vi "convert abs chan num.vi"(0 "Abs Channel":i32, 5 "error in":errorcluster) -> (12 "num channels":i32, 13 "num pages":i32, 14 "Card type":string, 15 "Slot num":i32, 16 "set page":i32, 17 "Channel number in card":i32, 18 "Crate Num":i32, 19 "error out":errorcluster)   [LabVIEW 2018]
uses:
  CAEN globals.vi
panel:
  out "Card num of type":i32
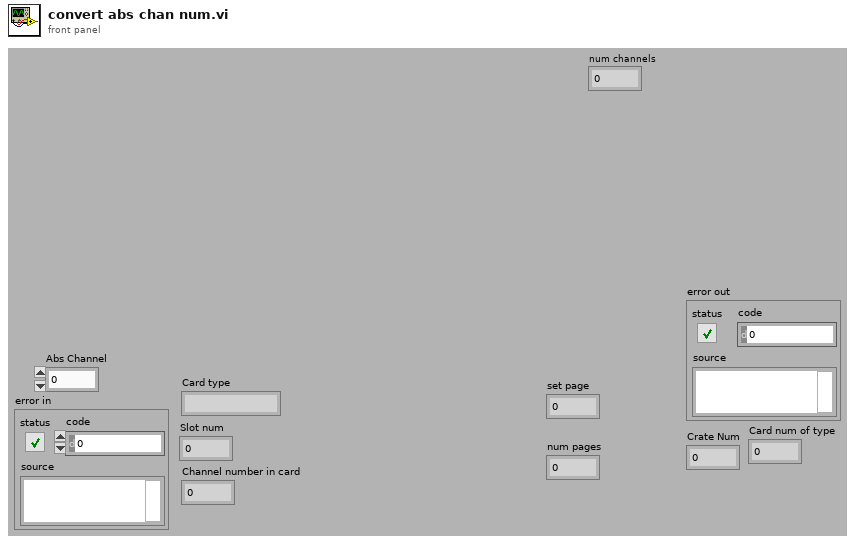
[diagram p1: front panel]
types:
  T1 = typedef "crate.ctl" = cluster{"CAENet Address":i32, "Crate Model":string, "Firmware Version":string, "Crate Map":T2[], "Total Channels":i32}
  T2 = typedef "card.ctl" = cluster{"Slot Number":i32, "Card Model":string, "Num Channels":i32, "Polarity":string, "Vmax":dbl, "Imax":dbl, "Revision":string}
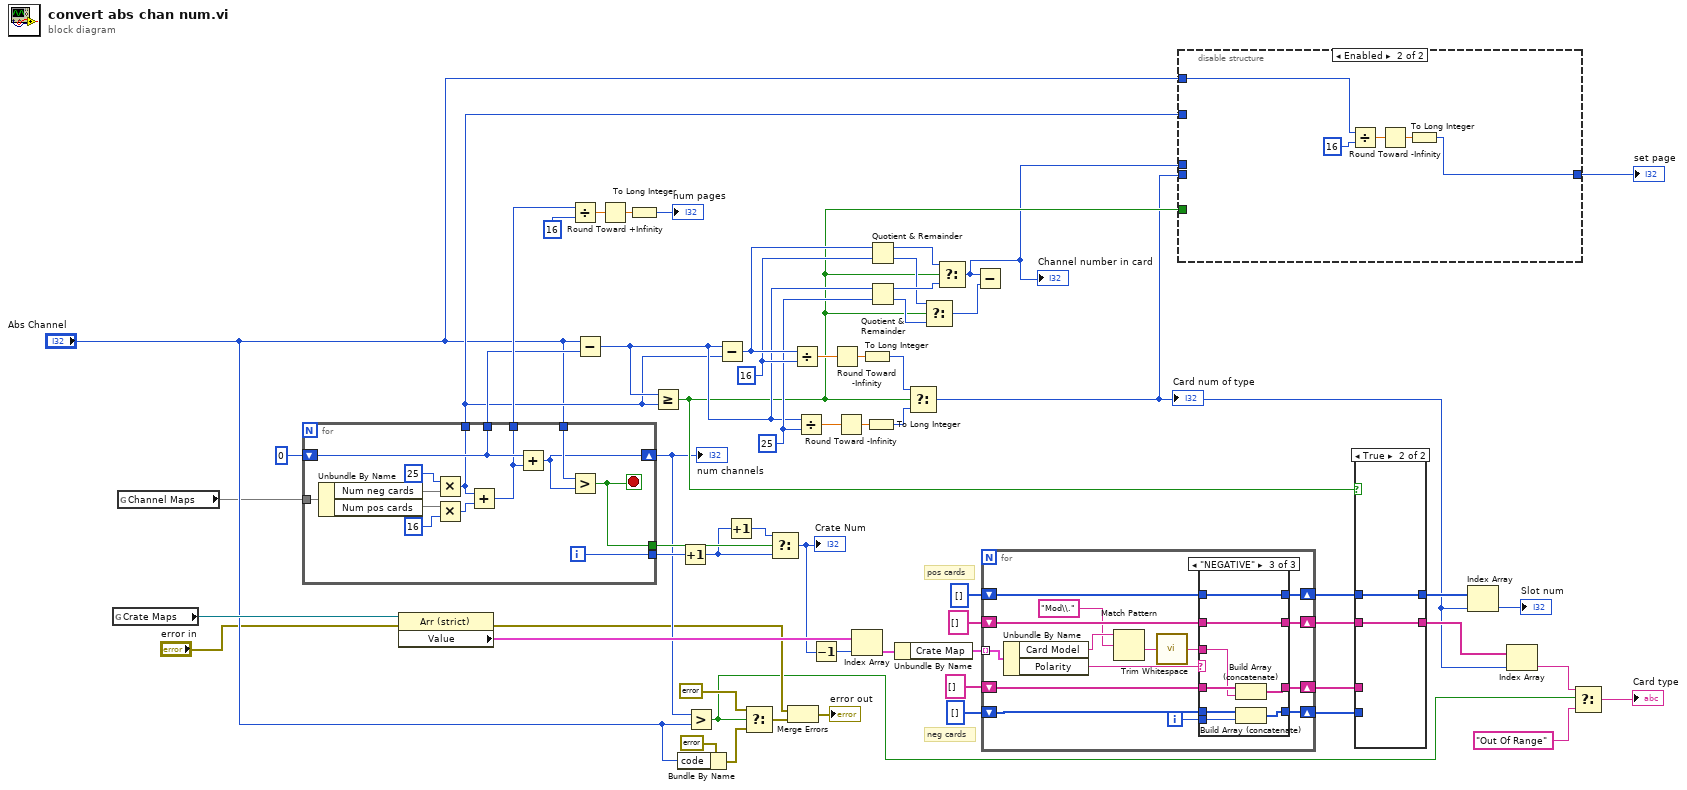
[diagram p0: block diagram]
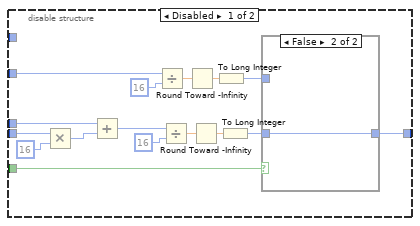
[diagram p2: hidden frame]
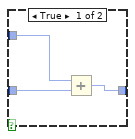
[diagram p3: hidden frame]
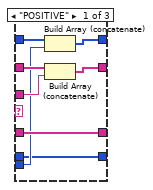
[diagram p5: hidden frame]
diagram:
  w54 = 25 ("y")
  w55 = 16 ("y")
  # "neg cards"
  # "pos cards"
  n1 = global read "CAEN globals.vi" "Crate Maps"() -> (w45:refnum<vi>)
  n2 = global read "CAEN globals.vi" "Channel Maps"() -> (w2)
  n3 = for {
    tunnel: w2 -> [w73]
    shift-right: [w68] -> w11
    shift-left: 0 -> [w67]
    tunnel: "Abs Channel" -> [w69]
    tunnel: [w65] -> w47
    tunnel: [w67] -> w20
    tunnel: [w66] -> w19
    tunnel: [w64] -> w49
    tunnel: [w63] -> w27
    i -> [w65]
    stop <- w64 stop-if-true
    n4 = Unbundle By Name(w73) -> ("Num neg cards"=w75, "Num pos cards"=w71)
    n5 = Multiply(x=25 ("y"), y=w75) -> (x*y=w66:i32)
    n6 = Multiply(x=w71, y=16) -> (x*y=w70:i32)
    n7 = Add(x=w66, y=w70) -> (x+y=w63:i32)
    n8 = Add(x=w67, y=w63) -> (x+y=w68:i32)
    n9 = Greater?(x=w69, y=w68) -> (0:w64:bool)
  }
  "num channels" <- w11
  n10 = property class="Arr (strict)"(reference=w45, error in="error in") -> (error out=w9:errorcluster, "Value"=w44:T1[])  [unwired: 1 out]
  n11 = Divide(x=w27, y=16) -> (x/y=w29:dbl)
  n12 = Subtract(x="Abs Channel", y=w20) -> (x-y=w51:i32)
  n13 = Round Toward +Infinity(x=w29) -> (ceil(x): smallest int >= x=w30:dbl)
  n14 = To Long Integer(number=w30) -> (32bit integer=→"num pages":i32)
  n15 = Greater Or Equal?(x=w51, y=w19) -> (x >= y?=w23:bool)
  n16 = Bundle By Name(cluster=errorcluster {"status"=TRUE, "code"=0, "source"="Channel out of range"} ("error out"), "code"="Abs Channel") -> (w15:errorcluster)
  n17 = Increment(x=w47) -> (x+1=w46:i32)
  n18 = Greater?(x=w11, y="Abs Channel") -> (0:w3:bool)
  n19 = Subtract(x=w51, y=w19) -> (x-y=w56:i32)
  n20 = Increment(x=w46) -> (x+1=w48:i32)
  n21 = Select(t=errorcluster {"status"=FALSE, "code"=0, "source"=""}, s=w3, f=w15) -> (s? t:f=w13:errorcluster)
  n22 = Select(t=w48, s=w49, f=w46) -> (s? t:f=w43:i32)
  "Crate Num" <- w43
  n23 = Merge Errors(w9, w13) -> (→"error out":errorcluster)
  n24 = Divide(x=w56, y=w55) -> (x/y=w57:dbl)
  n25 = Divide(x=w51, y=w54) -> (x/y=w61:dbl)
  n26 = Decrement(x=w43) -> (x-1=w42:i32)
  n27 = Round Toward -Infinity(1:w57) -> (0:w58:dbl)
  n28 = Round Toward -Infinity(1:w61) -> (0:w60:dbl)
  n29 = Index Array(array=w44, index=w42) -> (element=w41:T1)
  n30 = To Long Integer(number=w58) -> (32bit integer=w59:i32)
  n31 = To Long Integer(number=w60) -> (32bit integer=w62:i32)
  n32 = Quotient & Remainder(x=w56, y=w55) -> (x-y*floor(x/y)=w53:i32, floor(x/y)=w25:i32)
  n33 = Quotient & Remainder(x=w51, y=w54) -> (x-y*floor(x/y)=w52:i32, floor(x/y)=w24:i32)
  n34 = Unbundle By Name(w41) -> ("Crate Map"=w40:T2[])
  n35 = Select(t=w59, s=w23, f=w62) -> (s? t:f=w7:i32)
  "Card num of type" <- w7
  n36 = Select(t=w25, s=w23, f=w24) -> (s? t:f=w22:i32)
  n37 = Select(t=w53, s=w23, f=w52) -> (s? t:f=w21:i32)
  "Channel number in card" <- w21
  n38 = Subtract(x=w21, y=w22) -> ()  [unwired: 1 out]
  n39 = for {
    shift-right: [w86] -> w35
    shift-left: string[] [] -> [w89]
    shift-right: [w85] -> w33
    shift-left: string[] [] -> [w88]
    tunnel: w40 -> [w90] mode=indexing
    shift-right: [w76] -> w18
    shift-left: i32[] [] -> [w77]
    shift-right: [w78] -> w17
    shift-left: i32[] [] -> [w80]
    i -> [w79]
    n40 = Unbundle By Name(w90) -> ("Card Model"=w84:string, "Polarity"=w87:string)
    n41 = Match Pattern(string=w84, regular expression="Mod\\.") -> (after substring=w82:string)  [unwired: 1 in, 3 out]
    n42 = call <vilib>:"Trim Whitespace.vi"("string"=w82) -> ("trimmed string"=w81:string)  [unwired: 1 in]
    n43 = case shown="\"NEGATIVE\"" w87 {
      tunnel: w89 -> [w98 w102 w109]
      tunnel: w88 -> [w95 w101 w110]
      tunnel: w81 -> [w97 _ w108]
      tunnel: [w96 w102 w109] -> w86
      tunnel: [w95 w101 w107] -> w85
      tunnel: w80 -> [w91 w99 w106]
      tunnel: w79 -> [w93 _ w105]
      tunnel: [w91 w99 w104] -> w78
      tunnel: w77 -> [w94 w100 w103]
      tunnel: [w92 w100 w103] -> w76
      frame "POSITIVE" {
        n44 = Build Array (concatenate)(w94, w93) -> (w92:i32[])
        n45 = Build Array (concatenate)(w98, w97) -> (w96:string[])
      }
      frame "Not Present", Default {
      }
      frame "NEGATIVE" {
        n46 = Build Array (concatenate)(w110, w108) -> (w107:string[])
        n47 = Build Array (concatenate)(w106, w105) -> (w104:i32[])
      }
    }
  }
  n48 = disable-structure shown="Enabled" {
    disable-tunnel: w23 -> [w115 _]
    disable-tunnel: w19 -> [w114 _]
    disable-tunnel: w7 -> [w113 _]
    disable-tunnel: w21 -> [w112 _]
    disable-tunnel: [w111 w132] -> w26
    disable-tunnel: "Abs Channel" -> [_ w131]
    frame Disabled {
      n49 = Multiply(x=w113, y=16) -> (x*y=w126:i32)
      n50 = Add(x=w112, y=w126) -> (x+y=w117:i32)
      n51 = Divide(x=w114, y=16) -> (x/y=w122:dbl)
      n52 = Divide(x=w117, y=16) -> (x/y=w120:dbl)
      n53 = Round Toward -Infinity(1:w122) -> (0:w123:dbl)
      n54 = Round Toward -Infinity(1:w120) -> (0:w119:dbl)
      n55 = To Long Integer(number=w123) -> (32bit integer=w121:i32)
      n56 = To Long Integer(number=w119) -> (32bit integer=w116:i32)
      n57 = case shown="False" w115 {
        tunnel: [w129 w130] -> w111
        tunnel: w116 -> [w127 w130]
        tunnel: w121 -> [w128 _]
        frame True {
          n58 = Add(x=w128, y=w127) -> (x+y=w129:i32)
        }
        frame False {
        }
      }
    }
    frame Enabled {
      n59 = Divide(x=w131, y=16) -> (x/y=w133:dbl)
      n60 = Round Toward -Infinity(1:w133) -> (0:w134:dbl)
      n61 = To Long Integer(number=w134) -> (32bit integer=w132:i32)
    }
  }
  "set page" <- w26
  n62 = case shown="True" w23 {
    tunnel: [w136 w139] -> w34
    tunnel: w18 -> [_ w139]
    tunnel: [w137 w138] -> w8
    tunnel: w35 -> [_ w138]
    tunnel: w33 -> [w137 _]
    tunnel: w17 -> [w136 _]
    frame False {
    }
    frame True {
    }
  }
  n63 = Index Array(array=w34, index=w7) -> (element=→"Slot num":i32)
  n64 = Index Array(array=w8, index=w7) -> (element=w5:string)
  n65 = Select(t=w5, s=w3, f="Out Of Range") -> (s? t:f=→"Card type":string)
